vi "SF2 Get File List.vi"() -> ()   [LabVIEW 2016]
uses:
  <vilib>/Utility/file.llb/Read Delimited Spreadsheet (string).vi
panel:
  out "size(s)":i32[](array[numeric])
  out "Free Space (meg)":dbl
  out "File size (meg)":dbl
  out "all rows":string[][](array[string])
  out "filenames":string[](array[string])
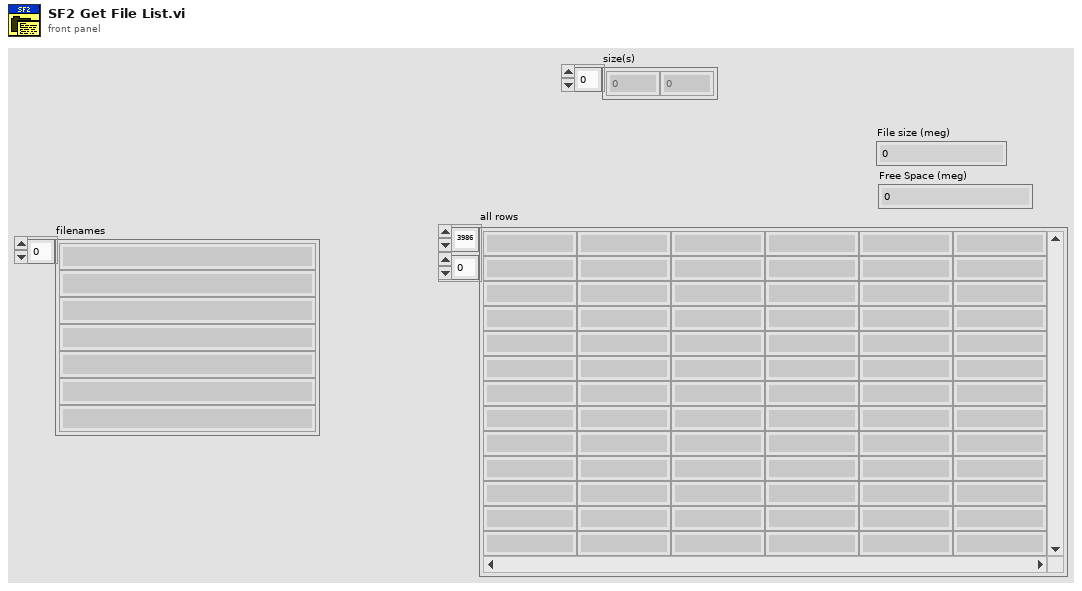
[diagram p1: front panel]
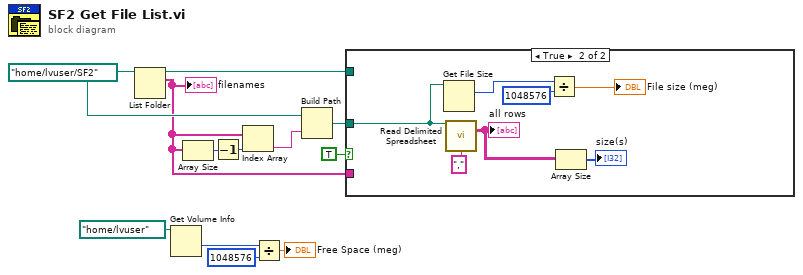
[diagram p0: block diagram]
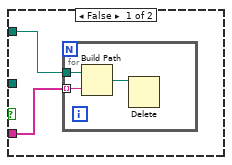
[diagram p2: hidden frame]
diagram:
  w7 = path "/home/lvuser/SF2" ("path (use dialog)")
  n1 = List Folder(path=w7) -> (filenames=w6:string[])  [unwired: 3 in, 3 out]
  "filenames" <- w6
  n2 = Get Volume Info(11:path "/home/lvuser" ("path (use dialog)")) -> (1:w3:i64)  [unwired: 1 in, 5 out]
  n3 = Array Size(array=w6) -> (size(s)=w11:i32)
  n4 = Decrement(x=w11) -> (x-1=w8:i32)
  n5 = Index Array(array=w6, index=w8) -> (element=w10:string)
  n6 = Divide(x=w3, y=i64 1048576) -> (x/y=→"Free Space (meg)":dbl)
  n7 = Build Path(base path=w7, name or relative path=w10) -> (appended path=w9:path)
  n8 = case shown="True" TRUE {
    tunnel: w9 -> [_ w22]
    tunnel: w7 -> [w13 _]
    tunnel: w6 -> [w12 _]
    frame False {
      n9 = for {
        tunnel: w13 -> [w16]
        tunnel: w12 -> [w15] mode=indexing
        n10 = Build Path(base path=w16, name or relative path=w15) -> (appended path=w14:path)
        n11 = Delete(path (use dialog)=w14) -> ()  [unwired: 4 in, 3 out]
      }
    }
    frame True {
      n12 = Get File Size(file=w22) -> (size (in bytes)=w20:i64)  [unwired: 1 in, 2 out]
      n13 = call-poly <vilib>:"Read Delimited Spreadsheet.vi"("file path (dialog if empty)"=w22, "delimiter (\\t)"="," ("delimiter (\\t)")) -> ("all rows"=w18:string[][])  [unwired: 8 in, 5 out]
      "all rows" <- w18
      n14 = Divide(x=w20, y=i64 1048576) -> (x/y=→"File size (meg)":dbl)
      n15 = Array Size(array=w18) -> (size(s)=→"size(s)":i32[])
    }
  }
